vi "Lower.vi"(8 "error in (no error)":errorcluster, 10 "Speed":dbl=-0.75 format="%#_13g", 11 "Gantry in":refnum<class "A3200.lvclass">) -> (0 "error out":errorcluster, 3 "Gantry out":refnum<class "A3200.lvclass">)   [LabVIEW 2016, in "A3200.lvclass"]
uses:
  A3200.lvclass
  A3200.lvclass/A3200.ctl
  <userlib>/Aerotech A3200.lnk/Motion/FreerunSingle.vi
  <userlib>/Aerotech A3200.lnk/Aerotech VIs.lvlib
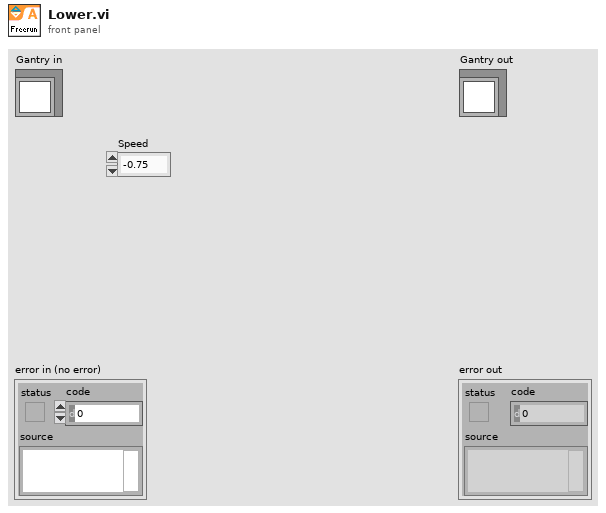
[diagram p1: front panel]
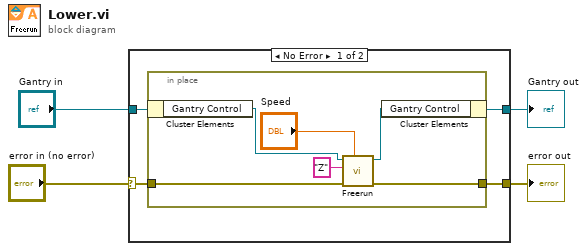
[diagram p0: block diagram]
diagram:
  n1 = case shown="No Error" "error in (no error)" {
    selector: "error in (no error)" -> [w6 w16]
    tunnel: "Gantry in" -> [w8 w15]
    tunnel: [w7 w15] -> w3
    tunnel: [w5 w16] -> w1
    frame No Error {
      n2 = in-place {
        in-place-border: w6 -> [w11]
        in-place-border: [w10] -> w5
        n3 = in-place-cluster #1(w8) -> ("Gantry Control"=w13:refnum<k24>)
        n4 = call-poly <userlib>:"Freerun.vi"("speed"="Speed", "error in (no error)"=w11, "axis name"="Z", "controller in"=w13) -> ("error out"=w10:errorcluster, "controller out"=w12:refnum<k24>)  [unwired: 6 in]
        n5 = in-place-cluster #1("Gantry Control"=w12) -> (w7:refnum<class "A3200.lvclass">)
      }
    }
    frame Error {
    }
  }
  "error out" <- w1
  "Gantry out" <- w3
